vi "F Dwf Enum Analog In Buffer Size.vi"(8 "error in (no error)":errorcluster, 10 "pnBufferSize":i32, 11 "idxDevice":i32) -> (0 "error out":errorcluster, 2 "pnBufferSize out":i32, 3 "function return":i32)   [LabVIEW 2019, in "Olasdwf.lvlib"]
doc: "DWFAPI int FDwfEnumAnalogInBufferSize(int idxDevice, int *pnBufferSize);"
uses:
  Olasdwf.lvlib
  Windows/System32/dwf.dll
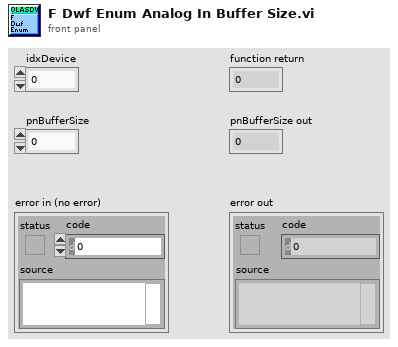
[diagram p1: front panel]
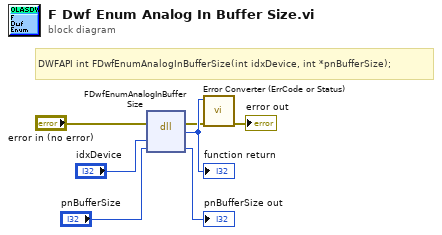
[diagram p0: block diagram]
diagram:
  # "DWFAPI int FDwfEnumAnalogInBufferSize(int idxDevice, int *pnBufferSize);"
  n1 = dll-call lib="C:/Windows/System32/dwf.*" fn="FDwfEnumAnalogInBufferSize"(error in="error in (no error)", "idxDevice"="idxDevice", "pnBufferSize"="pnBufferSize") -> (error out=w2:errorcluster, w7:i32, "pnBufferSize"=→"pnBufferSize out":i32)  [unwired: 3 in, 1 out]
  "function return" <- w7
  n2 = call "Error Converter (ErrCode or Status).vi"("error in (no error)"=w2, "error code"=w7) -> ("error out"=→"error out":errorcluster)  [unwired: 9 in]
